vi "Handle Last Ack Core.vi"(4 "error in (no error)":errorcluster, 6 "Last Ack":refnum<class "Last Ack.lvclass">, 7 "Child_5_Class in":refnum<class "Error_Emgime_Class.lvclass">) -> (0 "error out":errorcluster, 3 "Child_5_Class out":refnum<class "Error_Emgime_Class.lvclass">)   [LabVIEW 2023, in "Error_Engine_Actor.lvlib" / "Error_Emgime_Class.lvclass"]
doc: "(<B>Filename</B>: Actor Framework.lvlib:Actor.lvclass:Handle Last Ack Core.vi)\n\nDefines how the caller actor responds to the Last Ack message from a nested actor. The Last Ack message is the final message a nested actor sends to its caller before it shuts down. The message contains information about the final state of the nested actor.\n\nBy default, this method does nothing except return any error the nested actor sent. A descendant class may override this method to define behavior."
uses:
  Error_Emgime_Class.lvclass
  <vilib>/ActorFramework/LastAck/Last Ack.lvclass
  Abstraction_Interface_Class/Abstraction_Interface_Class.lvclass
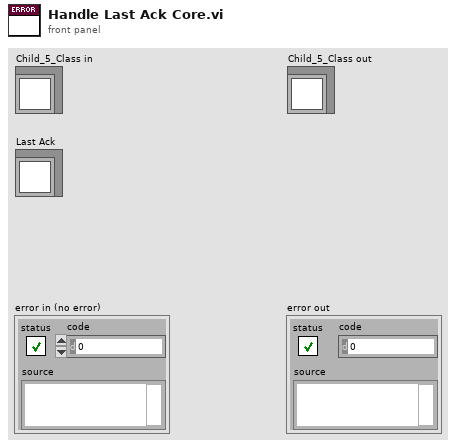
[diagram p1: front panel]
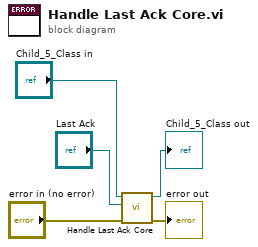
[diagram p0: block diagram]
diagram:
  n1 = call-parent "Handle Last Ack Core.vi"("error in (no error)"="error in (no error)", "Last Ack"="Last Ack", "Actor in"="Child_5_Class in") -> ("error out"=→"error out":errorcluster, "Actor out"=→"Child_5_Class out":refnum<class "Error_Emgime_Class.lvclass">)  [unwired: 3 in]
